vi "Seq count String.vi"(10 "dbl in":dbl) -> (2 "Int String Out":string)   [LabVIEW 2020, in "Controller.lvlib" / "Controller.lvclass"]
uses:
  Controller.lvclass
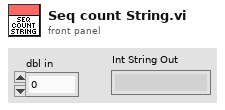
[diagram p1: front panel]
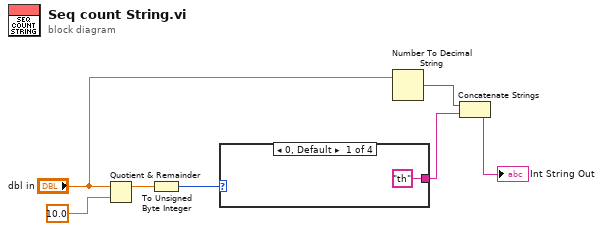
[diagram p0: block diagram]
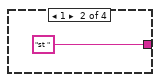
[diagram p2: hidden frame]
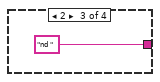
[diagram p3: hidden frame]
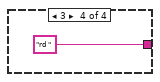
[diagram p4: hidden frame]
diagram:
  n1 = Quotient & Remainder(x="dbl in", y=10.0) -> (x-y*floor(x/y)=w6:dbl)  [unwired: 1 out]
  n2 = To Unsigned Byte Integer(number=w6) -> (unsigned 8bit integer=w5:u8)
  n3 = case shown="0, Default" w5 {
    tunnel: ["th" "st " "nd " "rd "] -> w2
    frame 0, Default {
    }
    frame 1 {
    }
    frame 2 {
    }
    frame 3 {
    }
  }
  n4 = Number To Decimal String(number="dbl in") -> (decimal integer string=w3:string)  [unwired: 1 in]
  n5 = Concatenate Strings(w3, w2) -> (→"Int String Out":string)
